vi "IsTransform.vi"(8 "error in (no error)":errorcluster, 11 "TransformTokenizer in":refnum<class "TransformTokenizer.lvclass">) -> (0 "error out":errorcluster, 2 "Transform?":bool, 3 "TransformTokenizer out":refnum<class "TransformTokenizer.lvclass">)   [LabVIEW 2019, in "TransformTokenizer.lvclass"]
uses:
  TransformTokenizer.lvclass
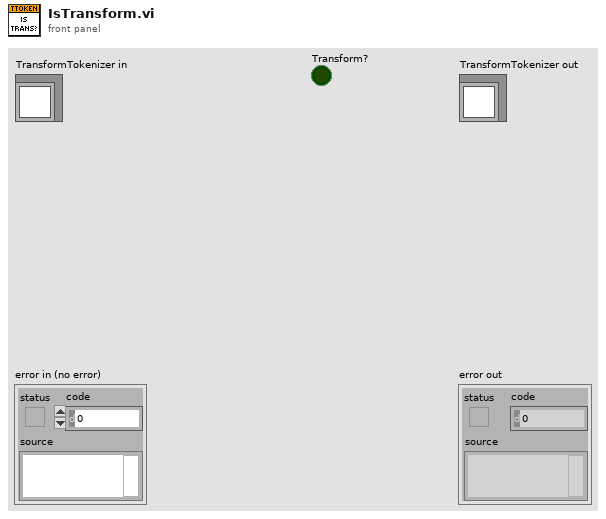
[diagram p1: front panel]
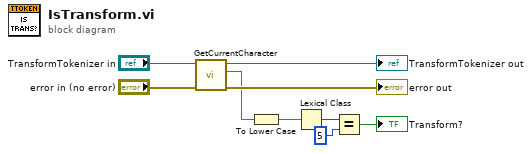
[diagram p0: block diagram]
diagram:
  n1 = call "GetCurrentCharacter.vi"("error in (no error)"="error in (no error)", "TransformTokenizer in"="TransformTokenizer in") -> ("error out"=→"error out":errorcluster, "Character"=w5:string, "TransformTokenizer out"=→"TransformTokenizer out":refnum<class "TransformTokenizer.lvclass">)  [unwired: 7 in]
  n2 = To Lower Case(string=w5) -> (all lower case string=w4:string)
  n3 = Lexical Class(1:w4) -> (0:w3:i16)
  n4 = Equal?(x=w3, y=i16 5) -> (x = y?=→"Transform?":bool)
